vi "find_special_character.vi"(8 "error in (no error)":errorcluster, 10 "Character":string, 11 "Command String":string) -> (0 "error out":errorcluster, 2 "Offset Array":i32[](array[numeric]))   [LabVIEW 2018]
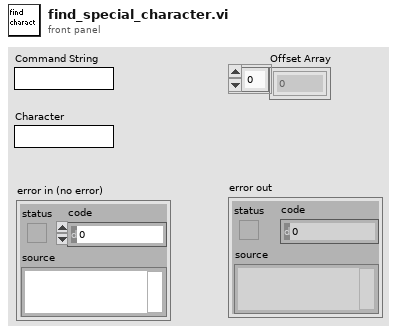
[diagram p1: front panel]
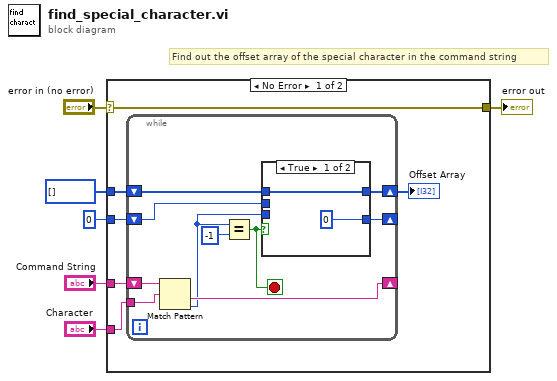
[diagram p0: block diagram]
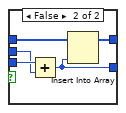
[diagram p2: hidden frame]
diagram:
  # "Find out the offset array of the special character in the command string"
  n1 = case shown="No Error" "error in (no error)" {
    selector: "error in (no error)" -> [w7 w30]
    tunnel: 0 ("y") -> [w11 _]
    tunnel: i32[] [] -> [w10 _]
    tunnel: "Command String" -> [w9 _]
    tunnel: "Character" -> [w8 _]
    tunnel: [w7 w30] -> w1
    frame No Error {
      n2 = while {
        tunnel: w8 -> [w21]
        shift-right: [w20] -> _
        shift-left: w9 -> [w22]
        shift-right: [w13] -> _
        shift-left: w11 -> [w14]
        shift-right: [w15] -> w12
        shift-left: w10 -> [w18]
        stop <- w17 stop-if-true
        n3 = Match Pattern(string=w22, regular expression=w21) -> (after substring=w20:string, offset past match=w16:i32)  [unwired: 3 out]
        n4 = Equal?(x=w16, y=-1) -> (x = y?=w17:bool)
        n5 = case shown="True" w17 {
          tunnel: w18 -> [w24 w29]
          tunnel: w16 -> [_ w27]
          tunnel: [w24 w28] -> w15
          tunnel: w14 -> [_ w26]
          tunnel: [0 w25] -> w13
          frame True {
          }
          frame False {
            n6 = Add(x=w27, y=w26) -> (x+y=w25:i32)
            n7 = Insert Into Array(array=w29, new element=w25) -> (w28:i32[])  [unwired: 1 in]
          }
        }
      }
      "Offset Array" <- w12
    }
    frame Error {
    }
  }
  "error out" <- w1
